vi "WinCI Get Provider Name.vi"(8 "error in (no error)":errorcluster) -> (0 "error out":errorcluster, 3 "provider name":string)   [LabVIEW 2020, in "NI_SCC_WinCI.lvlib"]
uses:
  <vilib>/SourceControl/Providers/WinCI/NI_SCC_WinCI.lvlib
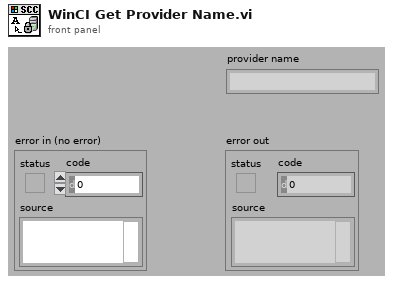
[diagram p1: front panel]
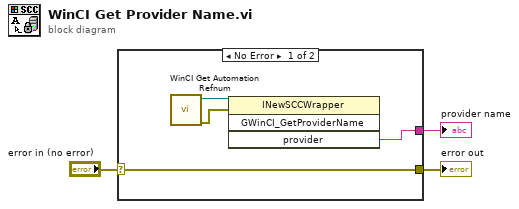
[diagram p0: block diagram]
diagram:
  n1 = case shown="No Error" "error in (no error)" {
    selector: "error in (no error)" -> [w7 w8]
    tunnel: [w7 w8] -> w2
    tunnel: [w6 _] -> w1
    frame No Error {
      n2 = call <vilib>:"WinCI Get Automation Refnum.vi"() -> ("error out"=w5:errorcluster, "automation refnum"=w4:refnum<k7>)  [unwired: 10 out]
      n3 = invoke class="INewSCCWrapper" method="GWinCI_GetProviderName"(reference=w4, error in=w5) -> ("provider"=w6:string)  [unwired: 2 in, 3 out]
    }
    frame Error {
    }
  }
  "error out" <- w2
  "provider name" <- w1
